vi "SystemConfigEditorV6.vi"(2 "error in":errorcluster) -> (0 "error out":errorcluster, 1 "FLImDAQ out":T1={"Digitizer 1"="", "Digitizer 2"="", "Channel"=enum."Channel 0", "trigger source"="VAL_EXTERNAL", "trigger level"=0.5, "trigger delay"=1.35e-07, "min sample rate"=12500000000.0, "min record length"=2500, "vertical range"=1.0, "vertical offset"=-0.25, "Waveform to Avg"=2000} {"trigger delay" format="%^#.4e"; "trigger level" format="%.4f"; "vertical offset" format="%.4f"; "vertical range" format="%.2f"; "min record length" format="%^#.4e"; "min sample rate" min=0.0 max=3.5 step=0.5 format="%.2f"})   [LabVIEW 2019]
uses:
  <userlib>/_OpenG.lib/file/file.llb/openg_file.lvlib
  <instrlib>/niScope/Controls/niScope trigger source.ctl
  FLImDAQ.ctl
panel:
  in  "FLImDAQ":T1={"Digitizer 1"="PXI1Slot3", "Digitizer 2"="PXI1Slot4", "Channel"=enum."Channel 0&1", "trigger source"="VAL_EXTERNAL", "trigger level"=0.5, "trigger delay"=2.5e-08, "min sample rate"=2500000000.0, "min record length"=600, "vertical range"=2.0, "vertical offset"=0.8, "Waveform to Avg"=4} caption="FLIm DAQ Configuration" {"trigger delay" format="%^#.4e"; "trigger level" min=0.0 max=3.5 step=0.5 format="%.2f"; "vertical offset" format="%.4f"; "vertical range" format="%.2f"; "min sample rate" format="%#.2p"}
  out "Configuration File Path":path
  in  "Confirm":bool
  in  "Load":bool
  in  "Save":bool
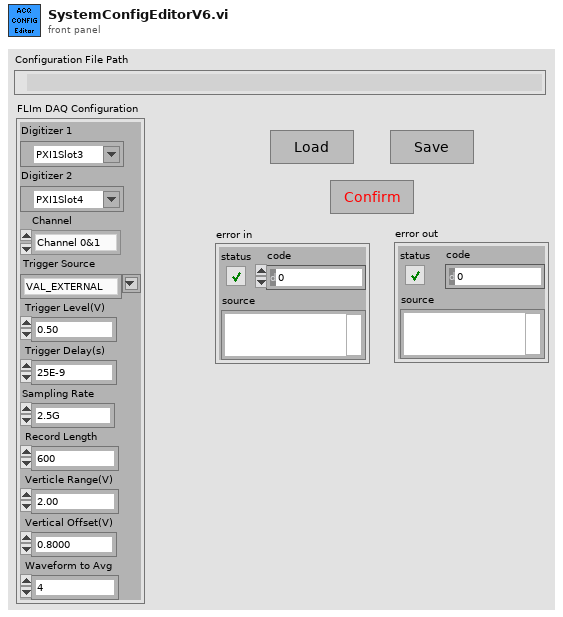
[diagram p1: front panel]
types:
  T1 = typedef "FLImDAQ.ctl" = cluster{"Digitizer 1":refnum<k15>, "Digitizer 2":refnum<k15>, "Channel":enum16{"Channel 0", "Channel 1", "Channel 0&1"}, "trigger source":T2, "trigger level":dbl, "trigger delay":dbl, "min sample rate":dbl, "min record length":i32, "vertical range":dbl, "vertical offset":dbl, "Waveform to Avg":i16}
  T2 = typedef "niScope trigger source.ctl" = string
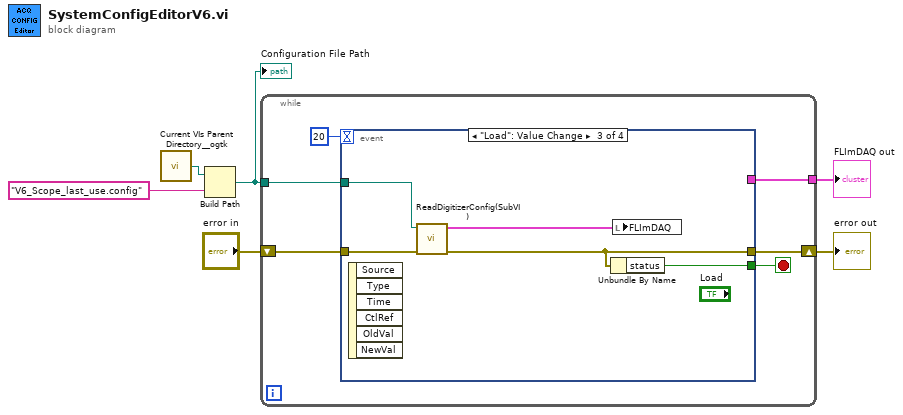
[diagram p0: block diagram]
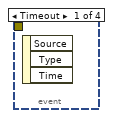
[diagram p2: hidden frame]
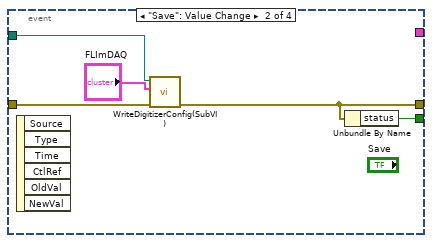
[diagram p3: hidden frame]
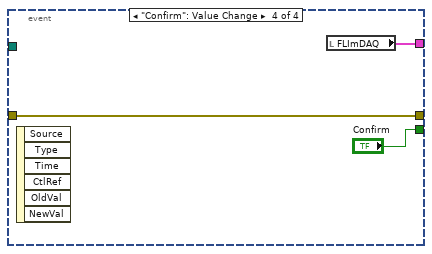
[diagram p4: hidden frame]
diagram:
  n1 = call <userlib>:"Current VIs Parent Directory__ogtk.vi"() -> ("Parent Directory (+ Relative)"=w5:path)  [unwired: 5 in]
  n2 = Build Path(base path=w5, name or relative path="V6_Scope_last_use.config") -> (appended path=w4:path)
  "Configuration File Path" <- w4
  n3 = while {
    tunnel: w4 -> [w10]
    shift-right: [w8] -> w3
    shift-left: "error in" -> [w9]
    tunnel: [w7] -> w1
    stop <- w11 stop-if-true
    n4 = event shown="[2] \"Load\": Value Change" {
      selector: _ -> [_ _ _ _]
      dyn-events: _ -> [_ _ _ _]
      timeout: 20 -> [_ _ _ _]
      tunnel: [_ w14 w18 "Confirm"] -> w11
      tunnel: w10 -> [_ w17 w22 _]
      tunnel: w9 -> [_ w16 w21 w24]
      tunnel: [_ w15 w19 w24] -> w8
      tunnel: [_ _ _ w23] -> w7
      event Timeout {
        n5 = event-data() -> ()  [unwired: 1 in, 3 out]
      }
      event "Save": Value Change {
        n6 = event-data() -> ()  [unwired: 1 in, 6 out]
        n7 = call "WriteDigitizerConfig(SubVI).vi"("error in (no error)"=w16, "FLImDAQ"="FLImDAQ", "appended path"=w17) -> ("error out"=w15:errorcluster)  [unwired: 8 in]
        n8 = Unbundle By Name(w15) -> ("status"=w14:bool)
      }
      event "Load": Value Change {
        n9 = event-data() -> ()  [unwired: 1 in, 6 out]
        n10 = call "ReadDigitizerConfig(SubVI).vi"("error in (no error)"=w21, "appended path"=w22) -> ("error out"=w19:errorcluster, "FLImDAQ"=w20:T1)  [unwired: 8 in]
        n11 = Unbundle By Name(w19) -> ("status"=w18:bool)
        n12 = local write "FLImDAQ"(w20) -> ()
      }
      event "Confirm": Value Change {
        n13 = event-data() -> ()  [unwired: 1 in, 6 out]
        n14 = local read "FLImDAQ"() -> (w23:T1)
      }
    }
  }
  "error out" <- w3
  "FLImDAQ out" <- w1
